vi "subDFD_Channel Simulation.vi"(11 "transmitted signal":cdb[](array[numeric]) format="%0.2f") -> (3 "recieved signal":cdb[](array[numeric]))   [LabVIEW 2023]
uses:
  <vilib>/Analysis/NI_AALBase.lvlib
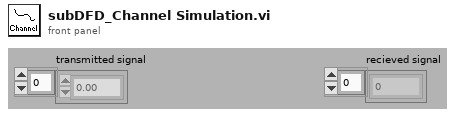
[diagram p1: front panel]
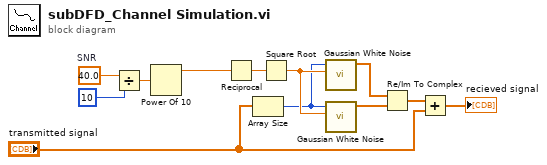
[diagram p0: block diagram]
diagram:
  w8 = 40.0  # SNR
  n1 = Divide(x=w8, y=10) -> (x/y=w12:dbl)
  n2 = Power Of 10(x=w12) -> (10^x=w10:dbl)
  n3 = Reciprocal(x=w10) -> (1/x=w9:dbl)
  n4 = Array Size(array="transmitted signal") -> (size(s)=w3:i32)
  n5 = Square Root(x=w9) -> (sqrt(x)=w7:dbl)
  n6 = call <vilib>:"Gaussian White Noise.vi"("standard deviation"=w7, "samples"=w3) -> ("Gaussian noise pattern"=w5:dbl[])  [unwired: 8 in, 1 out]
  n7 = call <vilib>:"Gaussian White Noise.vi"("standard deviation"=w7, "samples"=w3) -> ("Gaussian noise pattern"=w4:dbl[])  [unwired: 8 in, 1 out]
  n8 = Re/Im To Complex(1:w4, 2:w5) -> (0:w2:cdb[])
  n9 = Add(x=w2, y="transmitted signal") -> (x+y=→"recieved signal":cdb[])
